vi "Write Boolean Value.vi"(8 "error in (no error)":errorcluster, 10 "Boolean Value":bool, 11 "abs_Set_Boolean in":refnum<class "abs_Set_Boolean.lvclass">) -> (0 "error out":errorcluster, 3 "abs_Set_Boolean out":refnum<class "abs_Set_Boolean.lvclass">)   [LabVIEW 2021, in "BT.lvlib" / "abs_Set_Boolean.lvclass"]
uses:
  abs_Set_Boolean.lvclass
  abs_Set_Boolean.lvclass/abs_Set_Boolean.ctl
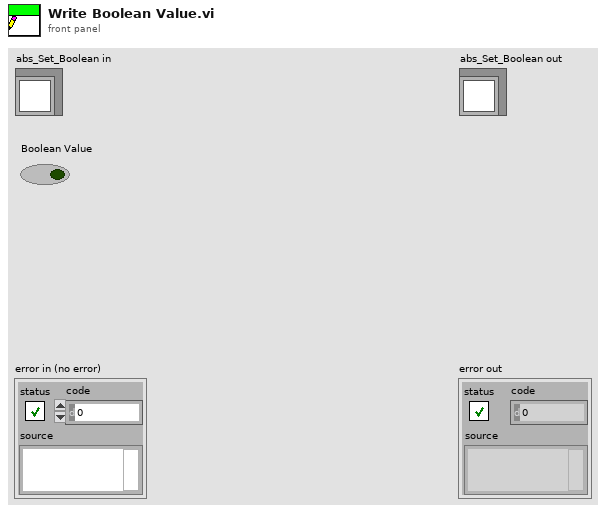
[diagram p1: front panel]
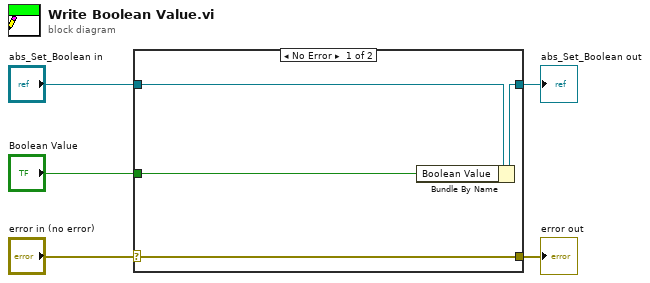
[diagram p0: block diagram]
diagram:
  n1 = case shown="No Error" "error in (no error)" {
    selector: "error in (no error)" -> [w9 w10]
    tunnel: [w9 w10] -> w4
    tunnel: [w7 w11] -> w2
    tunnel: "abs_Set_Boolean in" -> [w8 w11]
    tunnel: "Boolean Value" -> [w6 _]
    frame No Error {
      n2 = Bundle By Name(cluster=w8, "Boolean Value"=w6) -> (w7:refnum<class "abs_Set_Boolean.lvclass">)
    }
    frame Error {
    }
  }
  "error out" <- w4
  "abs_Set_Boolean out" <- w2
